vi "Task Stop.vi"(8 "error in (no error)":errorcluster, 11 "ChartGuiTask in":refnum<class "ChartGuiTask.lvclass">) -> (0 "error out":errorcluster, 3 "ChartGuiTask out":refnum<class "ChartGuiTask.lvclass">)   [LabVIEW 2020, in "VolatusDemo.lvlib" / "ChartGuiTask.lvclass"]
uses:
  ChartGuiTask.lvclass
  ChartGuiTask.lvclass/ChartGuiTask.ctl
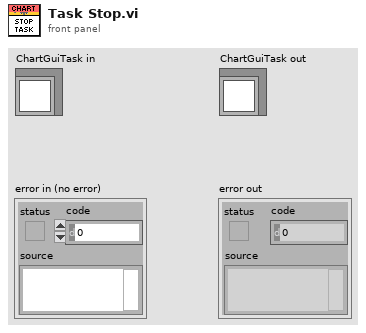
[diagram p1: front panel]
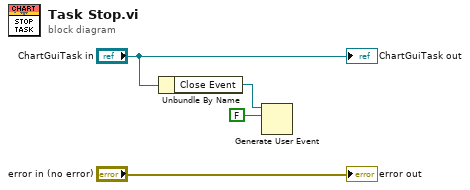
[diagram p0: block diagram]
diagram:
  n1 = Unbundle By Name("ChartGuiTask in") -> ("Close Event"=w2:refnum<user-event>)
  n2 = Generate User Event(user event=w2, event data cluster=FALSE ("event data")) -> ()  [unwired: 2 in, 2 out]
  "error out" <- "error in (no error)"
  "ChartGuiTask out" <- "ChartGuiTask in"
